vi "TeirToSensor.vi"(5 "Enum":T1) -> (0 "CL":dbl=0.35, 1 "CR":dbl=0.25, 2 "T1":dbl=0.42)   [LabVIEW 2014, in "Elevator System.lvlib"]
uses:
  Elevator System.lvlib
  Typedef/TeirNumber.ctl
panel:
  in  "CL":dbl=0.35 format="%#_13g"
  in  "Delta":dbl=0.84 format="%#_13g"
  in  "T1 Point":dbl=0.42 format="%#_13g"
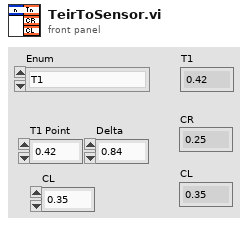
[diagram p1: front panel]
types:
  T1 = typedef "Elevator System.lvlib/TeirNumber.ctl" = enum16{"T1", "T2", "T3", "T4", "T5", "T6"}
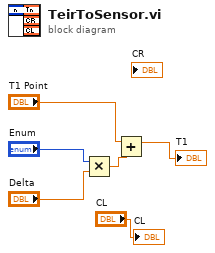
[diagram p0: block diagram]
diagram:
  n1 = Multiply(x="Enum", y="Delta") -> (x*y=w3:dbl)
  n2 = Add(x="T1 Point", y=w3) -> (x+y=→"T1":dbl)
  "CL" <- "CL"
